vi "phan - Copy.vi"() -> ()   [LabVIEW 2019]
uses:
  <vilib>/Platform/TimedLoop/XDataNode/timing_clust.ctl
  <vilib>/Platform/TimedLoop/XDataNode/nitl_modes.ctl
  <vilib>/Platform/TimedLoop/XDataNode/wakeup.ctl
  <vilib>/platform/TimedLoop/XDataNode/XDataNode.xnode
  <vilib>/Platform/TimedLoop/XDataNode/XDNodeRunTimeDep.lvlib
  <vilib>/ptbypt/NI_PtbyPt.lvlib
panel:
  in  "Kdv3":dbl
  in  "Kiv3":dbl=30.0
  in  "Kpv3":dbl=0.6
  in  "Kdv2":dbl
  in  "Kiv2":dbl=30.0
  in  "Kpv2":dbl=0.6
  in  "1000Ts":i64=200
  out "fs":dbl=10.0
  out "TOA DO 2":dbl[][](array[numeric])
  in  "fl":dbl=0.02 format="%0.3f"
  out "sailechS":cluster{"S":dbl, "Filtered x":dbl}(graph)
  in  "Kds":dbl
  in  "Kis":dbl
  in  "Kps":dbl=4.0
  in  "?":enum32{"DUONG HINH BUOM", "DUONGTRON"}(tab)
  in  "S_sp 2":dbl=0.13
  in  "R 2":dbl=0.5
  in  "phi_end 2":dbl=100.0
  in  "R":dbl=0.5
  in  "phi_end":dbl=100.0
  in  "phi_start":dbl=3.14 format="%#_13g"
  in  "S_sp":dbl=0.13
  out "V_ph":dbl
  out "V_dk":dbl
  out "w_ph3":dbl
  out "w_ph2":dbl
  out "w_ph1":dbl
  in  "RESETMAP":bool=TRUE caption="Reset"
  out "duty3":dbl
  out "duty2":dbl
  out "duty1":dbl
  in  "RESET":bool
  out "Y_sp":dbl
  out "X_sp":dbl
  out "Y_ph":dbl
  out "X_ph":dbl
  out "Map":cluster{"Y":dbl[], "Y":dbl[]}[](graph)
  out "V3_sp":dbl
  out "V3_ph":dbl
  out "VAN TOC":T1(graph)
  in  "Kdv1":dbl
  in  "Kiv1":dbl=30.0
  in  "Kpv1":dbl=0.6
  out "V2_ph":dbl
  out "V1_ph":dbl
  out "V2_sp":dbl
  out "V1_sp":dbl
  in  "START":bool
  # "HE THONG"
  # "PID VI TRI"
  # "PID TOC DO"
  # "DUTY"
  # "VI TRI DIEU KHIEN\n(m)"
  # "VI TRI PHAN HOI\n(m)"
  # "TOC DO PHAN HOI (rad/s)"
  # "VAN TOC DIEU KHIEN\n(m/s)"
  # "VAN TOC PHAN HOI\n(m/s)"
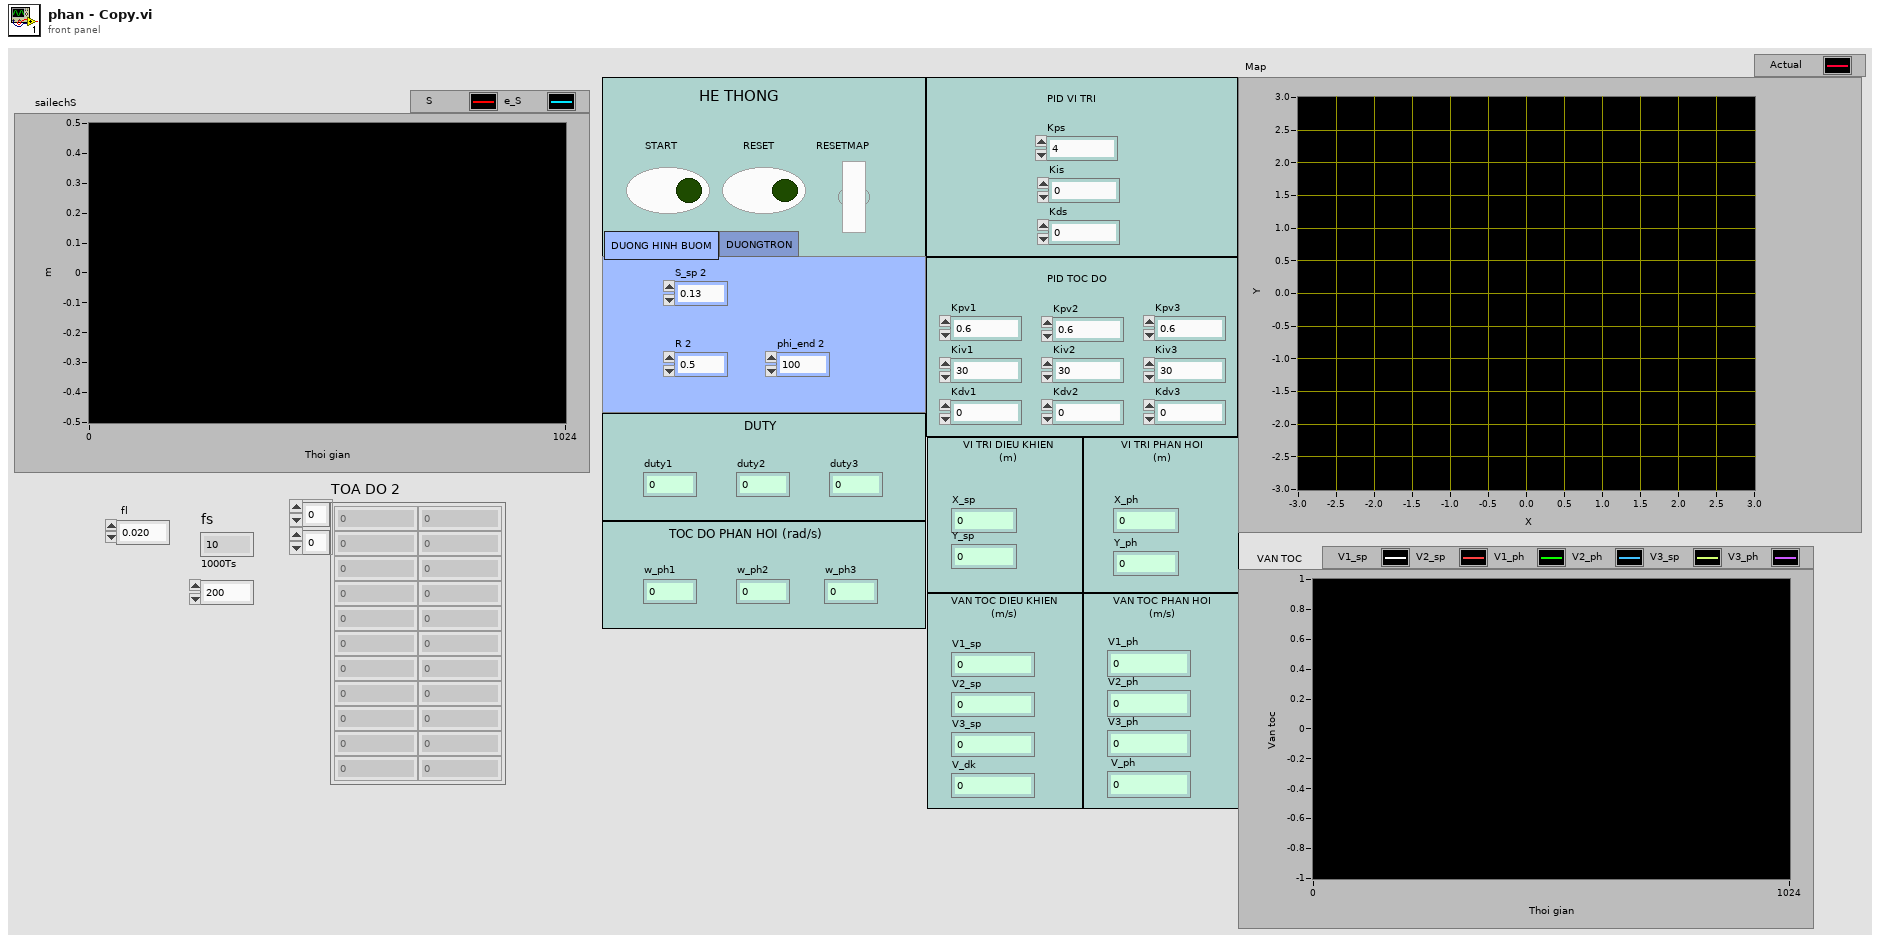
[diagram p1: front panel]
types:
  T1 = cluster{dbl, dbl, "V1_ph":dbl, "V2_ph":dbl, dbl, "V3_ph":dbl}
  T2 = typedef "XDNodeRunTimeDep.lvlib/timing_clust.ctl" = cluster{"Expected End [f-1]":u64, "Actual End [f-1]":u64, "Finished Late? [f-1]":bool, "Expected End [i-1]":u64, "Actual End [i-1]":u64, "Finished Late? [i-1]":bool, "Expected Start [i]":u64, "Actual Start [i]":u64, "Expected Start [f]":u64, "Actual Start [f]":u64, "Source Name":string, "Structure Name":string, "Period":i64, "Deadline":i64, "Offset":i64, "Start":i64, "Priority":i32, "Timeout":i32, "Mode":T3, "Wakeup Reason":T4, "Error":errorcluster, "Source Type":string, "Secondary Source Type":string, "Global End Time":u64, "Global Start Time":u64, "Frame Duration":u64, "Iteration Duration":u64, "Assigned CPU":i32, "I/O Scan Engine Mode":u32}
  T3 = typedef "XDNodeRunTimeDep.lvlib/nitl_modes.ctl" = enum32{"No Change", "Process missed periods, maintain original phase", "Discard missed periods, maintain original phase", "Process missed periods, ignore original phase", "Discard missed periods, ignore original phase"}
  T4 = typedef "XDNodeRunTimeDep.lvlib/wakeup.ctl" = enum32{"Normal", "Aborted", "Asynchronous wakeup", "Timing source error", "Timed loop error", "Timeout"}
  T5 = cluster{dbl, "V_ph1":dbl, dbl, "V_ph2":dbl, dbl, "V_ph3":dbl}
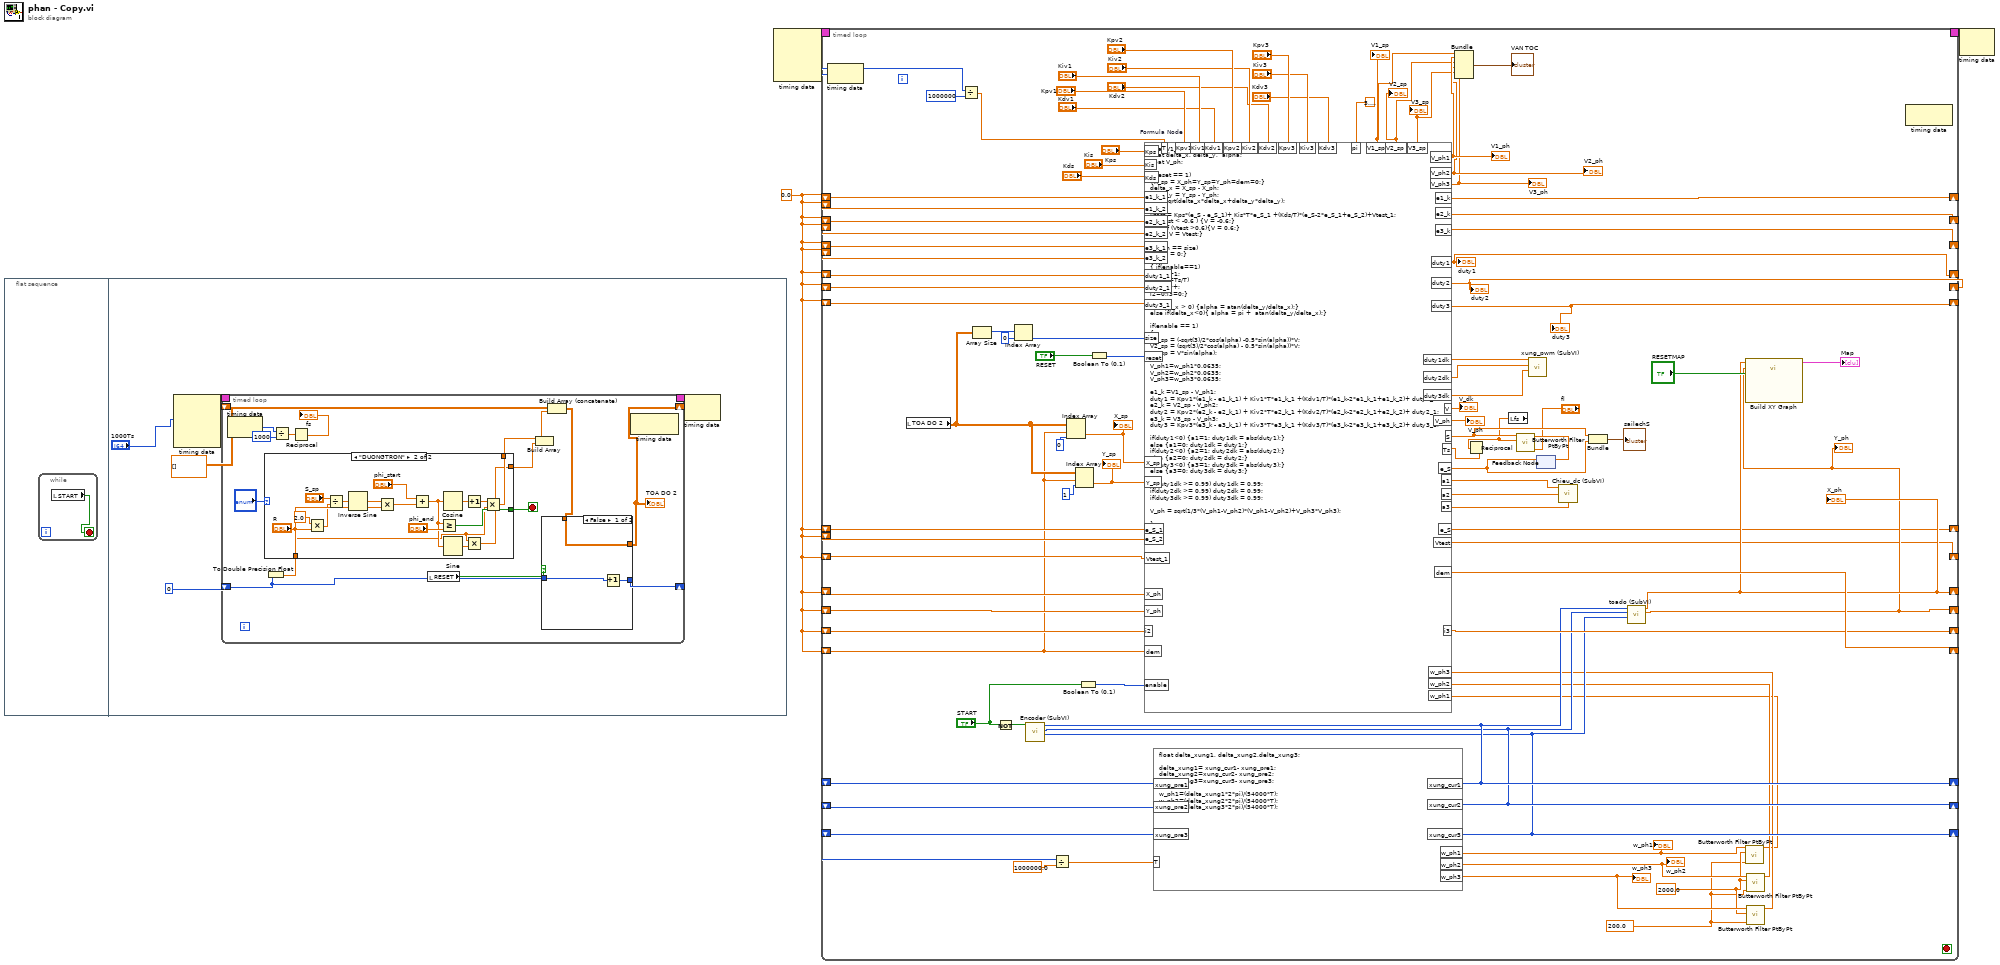
[diagram p0: block diagram]
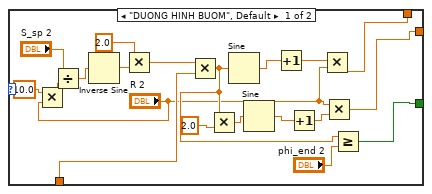
[diagram p2: hidden frame]
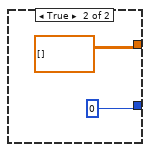
[diagram p3: hidden frame]
diagram:
  w1 = 0.0 ("e1")
  n1 = flat-sequence {
    frame #0 {
      n2 = while {
        stop <- w4 stop-if-true
        n3 = local read "START"() -> (w4:bool)
      }
    }
    frame #1 {
      n4 = node-c288("1000Ts") -> (w9:T2)  [unwired: 3 in]
      n5 = timed-loop {
        timing: w9 -> [_]
        timing-out: [_] -> w8
        shift-right: [w17] -> _
        shift-left: dbl[][] [] -> [w23]
        shift-right: [w21] -> _
        shift-left: 0 -> [w20]
        stop <- w12 stop-if-true
        n6 = node-c288() -> (w16:i64)  [unwired: 1 in]
        n7 = To Double Precision Float(number=w20) -> (double precision float=w25:dbl)
        n8 = case shown="\"DUONGTRON\"" "?" {
          tunnel: w25 -> [w45 w62]
          tunnel: [w37 w54] -> w19
          tunnel: [w38 w53] -> w18
          tunnel: [w34 w52] -> w12
          frame "DUONG HINH BUOM", Default {
            n9 = Multiply(x=10.0, y="R 2") -> (x*y=w32:dbl)
            n10 = Divide(x="S_sp 2", y=w32) -> (x/y=w29:dbl)
            n11 = Inverse Sine(1:w29) -> (0:w28:dbl)
            n12 = Multiply(x=2.0, y=w28) -> (x*y=w26:dbl)
            n13 = Multiply(x=w26, y=w45) -> (x*y=w35:dbl)
            n14 = Multiply(x=w35, y=2.0) -> (x*y=w40:dbl)
            n15 = Sine(x=w35) -> (sin(x)=w44:dbl)
            n16 = Sine(x=w40) -> (sin(x)=w41:dbl)
            n17 = Increment(x=w44) -> (x+1=w39:dbl)
            n18 = Increment(x=w41) -> (x+1=w42:dbl)
            n19 = Multiply(x=w39, y="R 2") -> (x*y=w37:dbl)
            n20 = Multiply(x="R 2", y=w42) -> (x*y=w38:dbl)
            n21 = Greater Or Equal?(x=w35, y="phi_end 2") -> (x >= y?=w34:bool)
          }
          frame "DUONGTRON" {
            n22 = Multiply(x=2.0, y="R") -> (x*y=w50:dbl)
            n23 = Divide(x="S_sp", y=w50) -> (x/y=w47:dbl)
            n24 = Inverse Sine(1:w47) -> (0:w46:dbl)
            n25 = Multiply(x=w46, y=w62) -> (x*y=w61:dbl)
            n26 = Add(x="phi_start", y=w61) -> (x+y=w58:dbl)
            n27 = Greater Or Equal?(x=w58, y="phi_end") -> (x >= y?=w52:bool)
            n28 = Cosine(x=w58) -> (cos(x)=w57:dbl)
            n29 = Sine(x=w58) -> (sin(x)=w55:dbl)
            n30 = Increment(x=w57) -> (x+1=w56:dbl)
            n31 = Multiply(x="R", y=w55) -> (x*y=w53:dbl)
            n32 = Multiply(x=w56, y="R") -> (x*y=w54:dbl)
          }
        }
        n33 = Divide(x=w16, y=i64 1000) -> (x/y=w14:dbl)
        n34 = Reciprocal(x=w14) -> (1/x=→"fs":dbl)
        n35 = local read "RESET"() -> (w11:bool)
        n36 = Build Array(w19, w18) -> (w24:dbl[])
        n37 = Build Array (concatenate)(w23, w24) -> (w22:dbl[][])
        n38 = case shown="False" w11 {
          tunnel: w22 -> [w65 _]
          tunnel: [w65 dbl[][] []] -> w17
          tunnel: [w64 0] -> w21
          tunnel: w20 -> [w63 _]
          frame False {
            n39 = Increment(x=w63) -> (x+1=w64:i32)
          }
          frame True {
          }
        }
        "TOA DO 2" <- w17
        n40 = node-c288() -> ()  [unwired: 1 in, 1 out]
      }
      n41 = node-c288(w8) -> ()  [unwired: 1 out]
    }
  }
  n42 = node-c288() -> (w3:T2)  [unwired: 4 in]
  n43 = timed-loop {
    timing: w3 -> [_]
    timing-out: [_] -> w2
    shift-right: [w171] -> _
    shift-left: w1 -> [w169]
    shift-right: [w170] -> _
    shift-left: w1 -> [w116]
    shift-right: [w162] -> _
    shift-left: w1 -> [w161]
    shift-right: [w139] -> _
    shift-left: w1 -> [w160]
    shift-right: [w138] -> _
    shift-left: w1 -> [w159]
    shift-right: [w158] -> _
    shift-left: w1 -> [w75]
    shift-right: [w136] -> _
    shift-left: w1 -> [w137]
    shift-right: [w135] -> _
    shift-left: w1 -> [w132]
    shift-right: [w134] -> _
    shift-left: w1 -> [w131]
    shift-right: [w133] -> _
    shift-left: w1 -> [w130]
    shift-right: [w119] -> _
    shift-left: _ -> [w127]
    shift-right: [w118] -> _
    shift-left: _ -> [w126]
    shift-right: [w117] -> _
    shift-left: _ -> [w125]
    shift-right: [w100] -> _
    shift-left: w1 -> [w110]
    shift-right: [w108] -> _
    shift-left: w1 -> [w109]
    shift-left: w1 -> [w104]
    shift-left: w1 -> [w103]
    shift-left: w1 -> [w102]
    shift-left: w1 -> [w101]
    stop <- _ stop-if-true
    w89 = 200.0 ("flw")
    w90 = 2000.0 ("sampling freq: fs")
    n44 = node-c288() -> (w122:i64)  [unwired: 1 in]
    n45 = local read "TOA DO 2"() -> (w76:dbl[][])
    n46 = Divide(x=w122, y=i64 1000000) -> (x/y=w120:dbl)
    n47 = Array Size(array=w76) -> (size(s)=w154:i32[])
    n48 = Not(x="START") -> (.not. x?=w141:bool)
    n49 = Index Array(array=w154, index=0) -> (element=w152:i32)
    n50 = call "Encoder (SubVI).vi"("Boolean"=w141) -> ("Counter Value3"=w117:i32, "Counter Value 2"=w118:i32, "Counter Value"=w119:i32)  [unwired: 8 in]
    n51 = Divide(x=w122, y=1000000.0) -> (x/y=w123:dbl)
    n52 = Index Array(array=w76, index (row)=w75, index (col)=0 ("disabled index (col)")) -> (element=w156:dbl)
    "X_sp" <- w156
    n53 = Index Array(array=w76, index (row)=w75, index (col)=1 ("disabled index (col)")) -> (element=w155:dbl)
    "Y_sp" <- w155
    n54 = Boolean To (0,1)(Boolean="START") -> (0, 1=w168:i16)
    n55 = Boolean To (0,1)(Boolean="RESET") -> (0, 1=w151:i16)
    n56 = formula code="float delta_xung1, delta_xung2,delta_xung3;\n\ndelta_xung1= xung_cur1- xung_pre1;\ndelta_xung2=xung_cur2- xung_pre2;\ndelta_xung3=xung_cur3- xung_pre3; \n\nw_ph1=(delta_xung1*2*pi)/(54000*T);\nw_ph2=(delta_xung2*2*pi)/(54000*T);\nw_ph3=(delta_xung3*2*pi)/(54000*T);"("xung_pre1"=w127, "xung_pre2"=w126, "xung_pre3"=w125, "xung_cur1"=w119, "xung_cur2"=w118, "xung_cur3"=w117, "T"=w123) -> ("w_ph1"=w78:dbl, "w_ph2"=w92:dbl, "w_ph3"=w91:dbl)
    "w_ph1" <- w78
    "w_ph2" <- w92
    "w_ph3" <- w91
    n57 = local read "fs"() -> (w86:dbl)
    n58 = Reciprocal(x=w86) -> (1/x=w85:dbl)
    n59 = feedback #1() -> (w97:dbl)  [unwired: 1 in]
    n60 = call "toado (SubVI).vi"("X3"=w117, "X2"=w118, "X1"=w119) -> ("Y_ph"=w138:dbl, "X_ph"=w139:dbl)  [unwired: 7 in]
    "X_ph" <- w139
    "Y_ph" <- w138
    n61 = call "Build XY Graph"("Reset"="RESETMAP", "Y Input"=w138, "X Input"=w139) -> ("XY Graph"=→"Map":cluster{"X":dbl[], "Y":dbl[]}[])  [unwired: 7 in, 1 out]
    n62 = call <vilib>:"Butterworth Filter PtByPt.vi"("low cutoff freq: fl"=w89, "sampling freq: fs"=w90, "x"=w78) -> ("Filtered x"=w77:dbl)  [unwired: 6 in, 1 out]
    n63 = call <vilib>:"Butterworth Filter PtByPt.vi"("low cutoff freq: fl"=w89, "sampling freq: fs"=w90, "x"=w92) -> ("Filtered x"=w88:dbl)  [unwired: 6 in, 1 out]
    n64 = call <vilib>:"Butterworth Filter PtByPt.vi"("low cutoff freq: fl"=w89, "sampling freq: fs"=w90, "x"=w91) -> ("Filtered x"=w87:dbl)  [unwired: 6 in, 1 out]
    n65 = formula code="float V1_sp, V2_sp,  V3_sp,V,Vtest;\nfloat delta_x, delta_y,  alpha;\nfloat V_ph;\n \nif(reset == 1)\n{X_sp = X_ph=Y_sp=Y_ph=dem=0;}\ndelta_x = X_sp - X_ph;\ndelta_y = Y_sp - Y_ph;\n S = sqrt(delta_x*delta_x+delta_y*delta_y); \n\nVtest = Kps*(e_S - e_S_1)+ Kis*T*e_S_1 +(Kds/T)*(e_S-2*e_S_1+e_S_2)+Vtest_1;\nif (Vtest < -0.6 ) {V = -0.6;} \nelse if (Vtest >0.6){V = 0.6;}\nelse {V = Vtest;}\n\nif(dem == size)\n{dem = 0;}\nelse\n{ if(enable==1)\n i3=i2+1;\nif (i3>=Ts/T)\n{dem++;\ni2=0;i3=0;}\n\nif(delta_x > 0) {alpha = atan(delta_y/delta_x);}\nelse if(delta_x<0){ alpha = pi +  atan(delta_y/delta_x);}\n\nif(enable == 1)\n{\nV1_sp = (-sqrt(3)/2*cos(alpha) -0.5*sin(alpha))*V;\nV2_sp = (sqrt(3)/2*cos(alpha) - 0.5*sin(alpha))*V;\nV3_sp = V*sin(alpha); \n\nV_ph1=w_ph1*0.0635;\nV_ph2=w_ph2*0.0635;\nV_ph3=w_ph3*0.0635;\n\ne1_k =V1_sp - V_ph1;\nduty1 = Kpv1*(e1_k - e1_k_1) + Kiv1*T*e1_k_1 +(Kdv1/T)*(e1_k-2*e1_k_1+e1_k_2)+ duty1_1;\ne2_k = V2_sp - V_ph2;\nduty2 = Kpv2*(e2_k - e2_k_1) + Kiv2*T*e2_k_1 +(Kdv2/T)*(e2_k-2*e2_k_1+e2_k_2)+ duty2_1;\ne3_k = V3_sp - V_ph3;\nduty3 = Kpv3*(e3_k - e3_k_1) + Kiv3*T*e3_k_1 +(Kdv3/T)*(e3_k-2*e3_k_1+e3_k_2)+ duty3_1;\n\nif(duty1<0) {a1=1; duty1dk = abs(duty1);}\nelse {a1=0; duty1dk = duty1;}\nif(duty2<0) {a2=1; duty2dk = abs(duty2);}\nelse {a2=0; duty2dk = duty2;}\nif(duty3<0) {a3=1; duty3dk = abs(duty3);}\nelse {a3=0; duty3dk = duty3;}\n\nif(duty1dk >= 0.99) duty1dk = 0.99;\nif(duty2dk >= 0.99) duty2dk = 0.99;\nif(duty3dk >= 0.99) duty3dk = 0.99;\n\nV_ph = sqrt(1/3*(V_ph1-V_ph2)*(V_ph1-V_ph2)+V_ph3*V_ph3);\n\n}\n}"("Kpv1"="Kpv1", "Kiv1"="Kiv1", "Kdv1"="Kdv1", "pi"=3.141592653589793, "e1_k_1"=w169, "e2_k_1"=w116, "enable"=w168, "T"=w120, "e3_k_1"=w161, "X_ph"=w160, "X_sp"=w156, "Y_sp"=w155, "Y_ph"=w159, "dem"=w75, "size"=w152, "reset"=w151, "i2"=w137, "duty1_1"=w132, "duty2_1"=w131, "duty3_1"=w130, "w_ph1"=w77, "w_ph2"=w88, "w_ph3"=w87, "e_S_1"=w110, "Vtest_1"=w109, "Kps"="Kps", "Kis"="Kis", "Kds"="Kds", "e1_k_2"=w104, "e2_k_2"=w103, "e3_k_2"=w102, "e_S_2"=w101, "e_S"=w97, "Ts"=w85, "Kpv2"="Kpv2", "Kiv2"="Kiv2", "Kdv2"="Kdv2", "Kpv3"="Kpv3", "Kiv3"="Kiv3", "Kdv3"="Kdv3") -> ("V1_sp"=w149:dbl, "V_ph1"=w148:dbl, "V_ph2"=w146:dbl, "e1_k"=w171:dbl, "e2_k"=w170:dbl, "V2_sp"=w147:dbl, "duty1"=w135:dbl, "duty2"=w134:dbl, "e3_k"=w162:dbl, "V_ph3"=w145:dbl, "V3_sp"=w144:dbl, "duty3"=w133:dbl, "a1"=w140:dbl, "a2"=w129:dbl, "a3"=w128:dbl, "dem"=w158:dbl, "i3"=w136:dbl, "duty1dk"=w115:dbl, "duty2dk"=w114:dbl, "duty3dk"=w113:dbl, "V"=→"V_dk":dbl, "V_ph"=→"V_ph":dbl, "e_S"=w100:dbl, "Vtest"=w108:dbl, "S"=w98:dbl)
    "V1_sp" <- w149
    "V2_sp" <- w147
    "V1_ph" <- w148
    "V2_ph" <- w146
    "V3_ph" <- w145
    "V3_sp" <- w144
    "duty1" <- w135
    "duty2" <- w134
    "duty3" <- w133
    n66 = Bundle(w149, "V_ph1"=w148, w147, "V_ph2"=w146, w144, "V_ph3"=w145) -> (→"VAN TOC":T5)  [unwired: 1 in]
    n67 = call <vilib>:"Butterworth Filter PtByPt.vi"("low cutoff freq: fl"="fl", "sampling freq: fs"=w86, "x"=w98) -> ("Filtered x"=w99:dbl)  [unwired: 6 in, 1 out]
    n68 = call "xung_pwm (SubVI).vi"("duty3 in"=w113, "duty2 in"=w114, "duty1 in"=w115) -> ()  [unwired: 6 in, 3 out]
    n69 = feedback-in #1(w99) -> ()
    n70 = call "Chieu_dc (SubVI).vi"("a3"=w128, "a2"=w129, "a1"=w140) -> ()
    n71 = Bundle("S"=w98, "Filtered x"=w97) -> (→"sailechS":cluster{"S":dbl, "Filtered x":dbl})  [unwired: 1 in]
    n72 = node-c288() -> ()  [unwired: 1 in, 1 out]
  }
  n73 = node-c288(w2) -> ()  [unwired: 1 out]
